vi "Ping.vi"(6 "timeout (ms)":i32=5000, 8 "error in":errorcluster, 11 "gRPC ID in":T4) -> (0 "error out":errorcluster, 2 "Loader Status":T1, 3 "gRPC ID out":T4)   [LabVIEW 2021, in "CIFPluginLoaderClientWrapper.lvlib"]
uses:
  CIFPluginLoaderClientWrapper.lvlib
  <vilib>/gRPC/LabVIEW gRPC Library/Shared/grpcId.ctl
  CIF_PluginLoader_client/RPC Messages/cif_manager_LoaderStatus.ctl
  CIF_PluginLoader_client/RPC Messages/cif_manager_LoaderInfo.ctl
  CIF_PluginLoader_client/RPC Messages/cif_manager_LoaderType.ctl
  CIF_PluginLoader_client/RPC Messages/cif_common_Empty.ctl
  CIF_PluginLoader_client/CIF_PluginLoader_client.lvlib
  <vilib>/gRPC/LabVIEW gRPC Library/grpc-lvsupport-release.lvlib
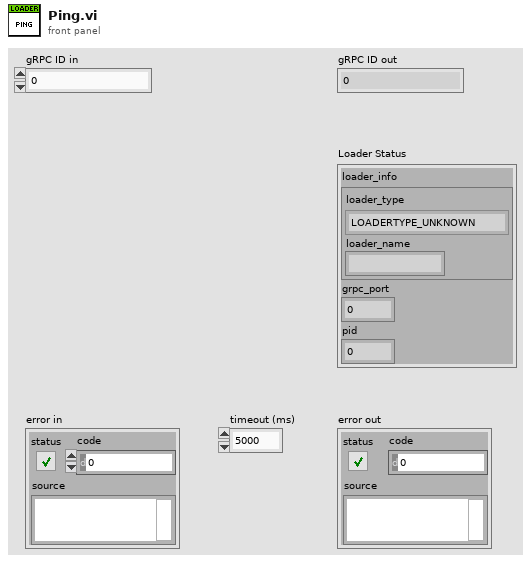
[diagram p1: front panel]
types:
  T1 = typedef "CIF_PluginLoader_client.lvlib/cif_manager_LoaderStatus.ctl" = cluster{"loader_info":T2, "grpc_port":i32, "pid":u32}
  T2 = typedef "CIF_PluginLoader_client.lvlib/cif_manager_LoaderInfo.ctl" = cluster{"loader_type":T3, "loader_name":string}
  T3 = typedef "CIF_PluginLoader_client.lvlib/cif_manager_LoaderType.ctl" = enum32{"LOADERTYPE_UNKNOWN", "LOADERTYPE_LABVIEW"}
  T4 = typedef "grpc-lvsupport-release.lvlib/grpcId.ctl" = u64
  T5 = typedef "CIF_PluginLoader_client.lvlib/cif_common_Empty.ctl" = cluster{"void":string}
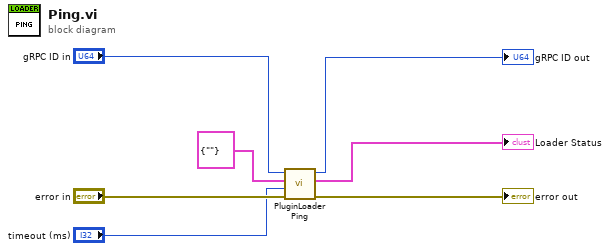
[diagram p0: block diagram]
diagram:
  n1 = call "PluginLoader Ping.vi"("error in"="error in", "timeout (ms)"="timeout (ms)", "Request Data"=T5 {"void"=""}, "gRPC ID"="gRPC ID in") -> ("error out"=→"error out":errorcluster, "Response Data"=→"Loader Status":T1, "gRPC ID out"=→"gRPC ID out":T4)  [unwired: 5 in]
